vi "Convert API String Arguments to Data(variant).vi"(7 "Type":variant, 9 "error in (no error)":errorcluster, 11 "String":string) -> (1 "error":errorcluster, 3 "Data":variant)   [LabVIEW 2017, in "API String Arguments Support.lvlib"]
uses:
  API String Arguments Support.lvlib
  <vilib>/Utility/Data Type/Type Definitions/Data Type.ctl
  <userlib>/_NEVSTOP/Communicable State Machine(CSM)/AdvanceAPI/CSM - Keywords.vi
  <userlib>/_OpenG.lib/string/string.llb/Trim Whitespace (String Array)__ogtk.vi
  <vilib>/Utility/Data Type/NI_Data Type.lvlib
  <userlib>/_NEVSTOP/Communicable State Machine(CSM)/Communicable State Machine.lvlib
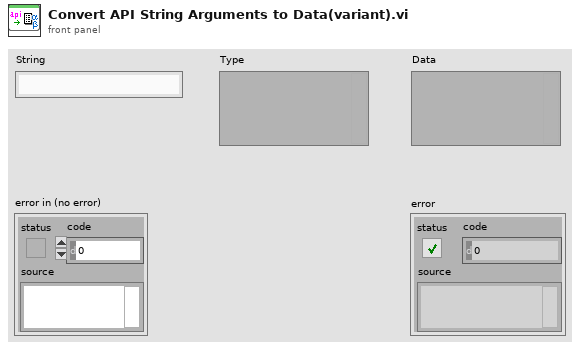
[diagram p1: front panel]
types:
  T1 = typedef "NI_Data Type.lvlib/Data Type.ctl" = enum8{"Invalid Type", "Void", "I8", "I16", "I32", "I64", "U8", "U16", "U32", "U64", "Single Float", "Double Float", "Extended Float", "Single Complex", "Double Complex", "Extended Complex", "Enum U8", "Enum U16", "Enum U32", "Enum U64", "Single Float With Unit", "Double Float With Unit", "Extended Float With Unit", "Single Complex with Unit", "Double Complex with Unit", "Extended Complex with Unit", "Boolean", "String", "Path", "Picture", "Tag", "Array", "Cluster", "Variant", "LV Variant", "Waveform", "Timestamp", "Digital Waveform", "Digital Data", "ExpressData", "Refnum", "External Data", "VI", "Poly VI", "LabVIEW Class Instance", "Fixed Point"}
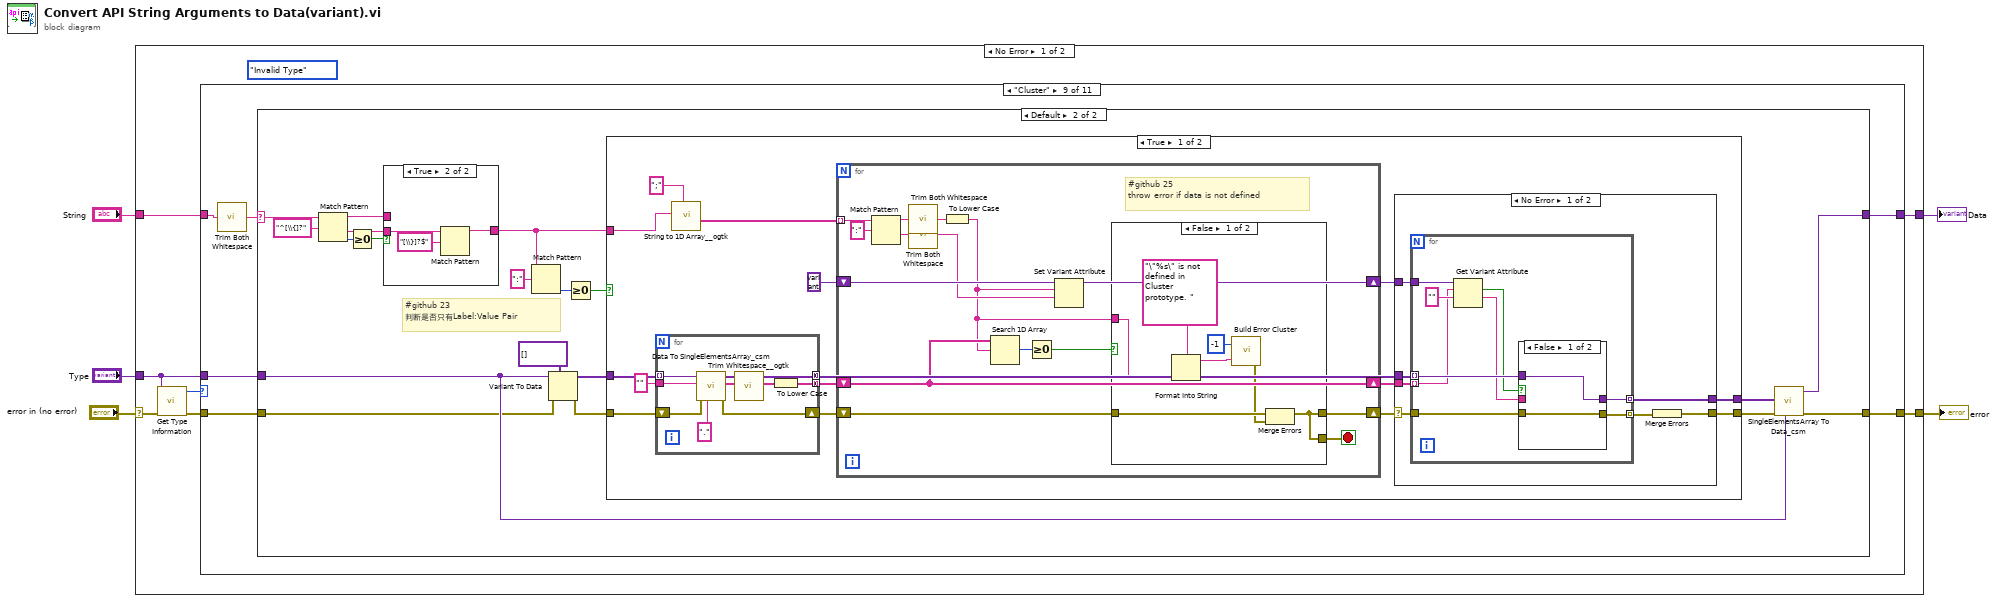
[diagram p0: block diagram]
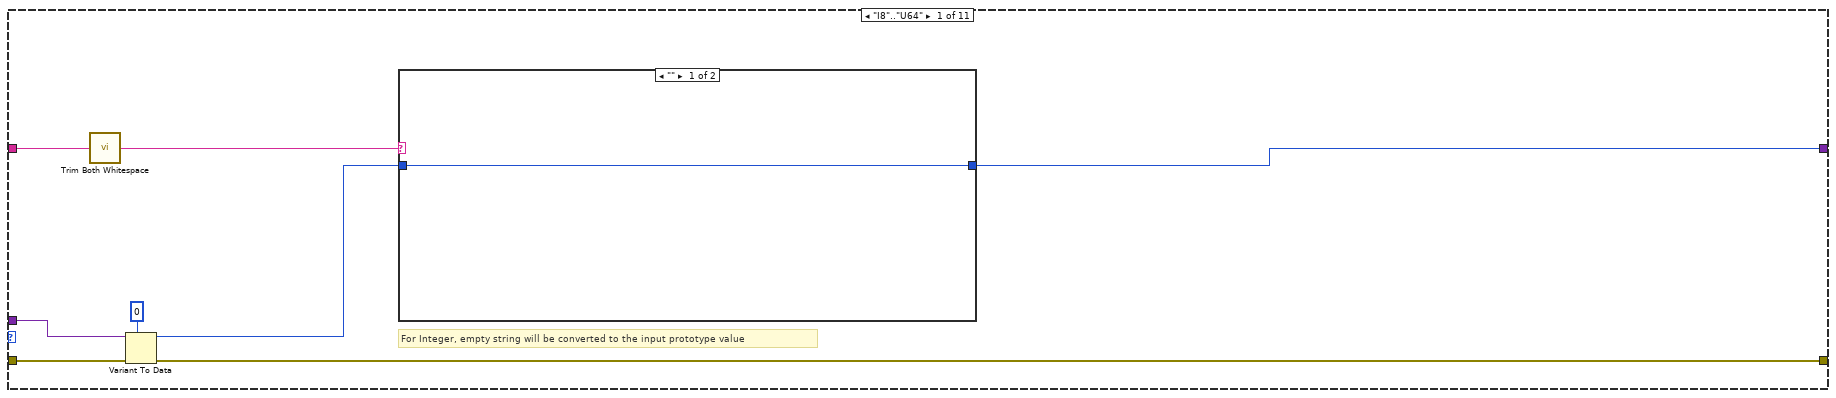
[diagram p2: hidden frame]
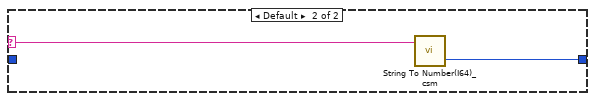
[diagram p3: hidden frame]
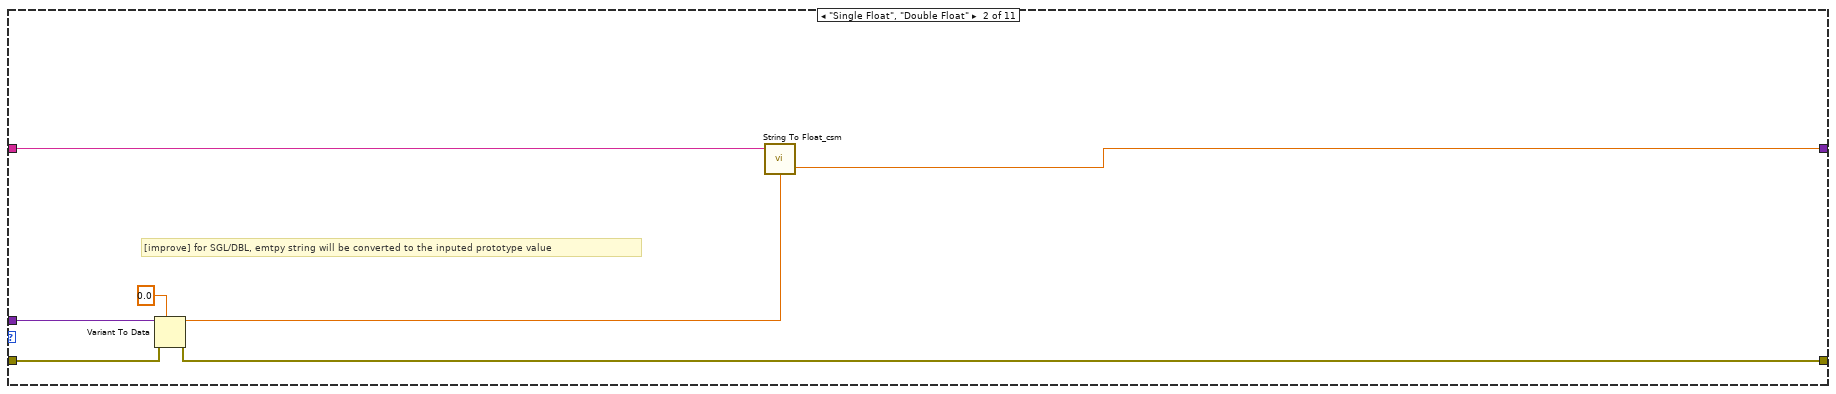
[diagram p4: hidden frame]
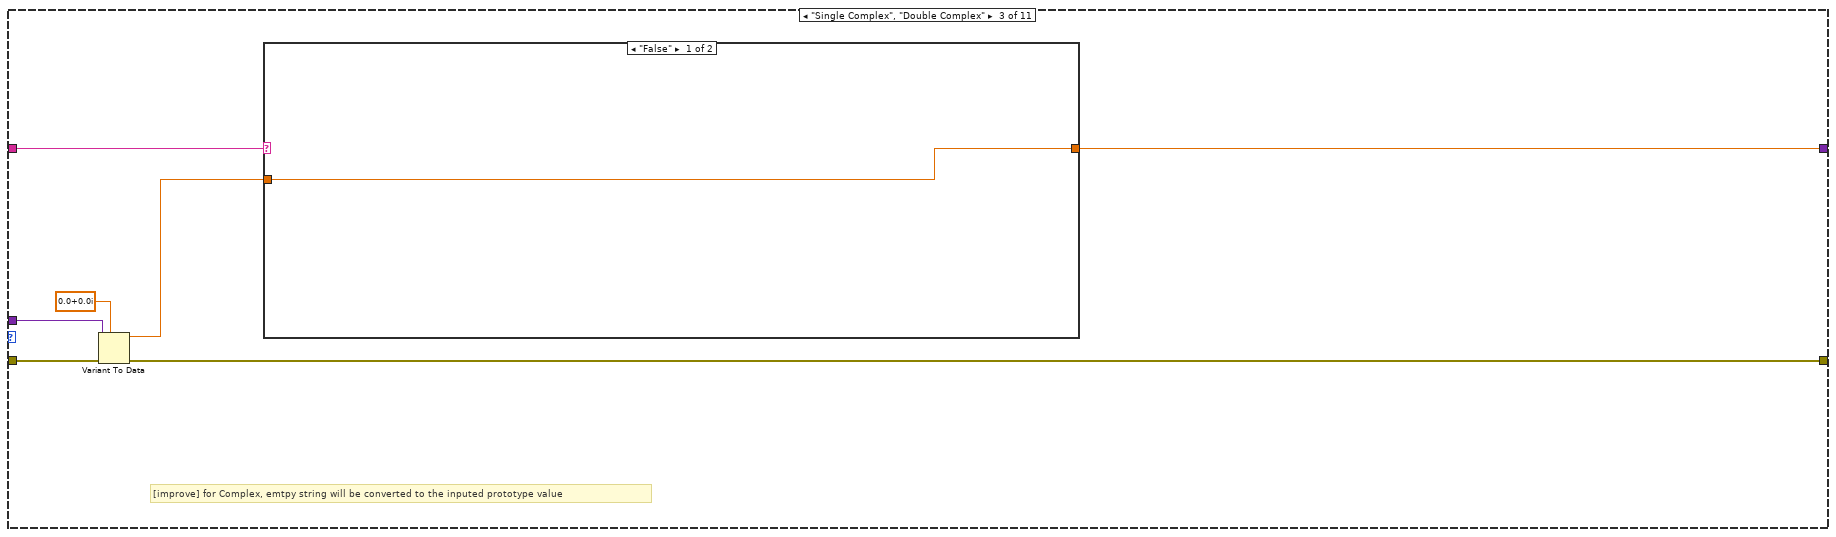
[diagram p5: hidden frame]
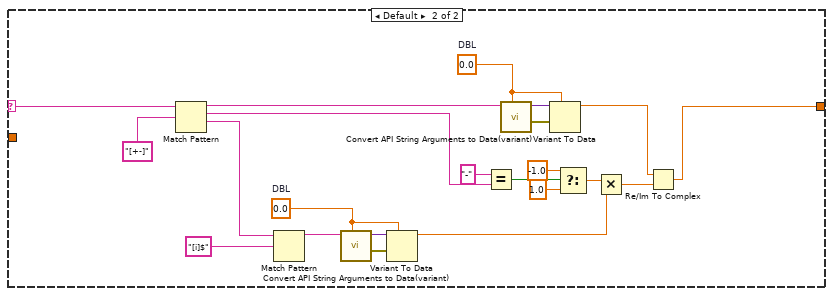
[diagram p6: hidden frame]
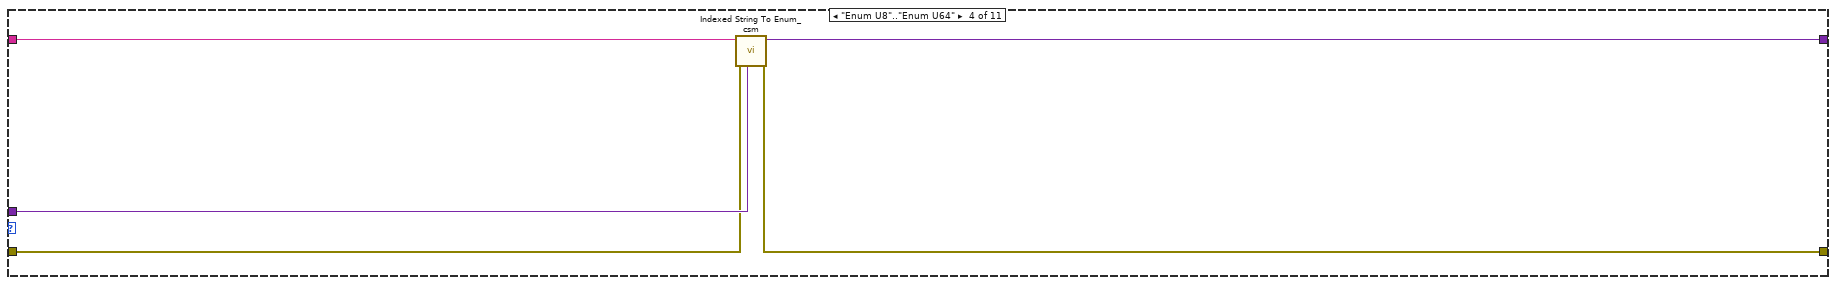
[diagram p7: hidden frame]
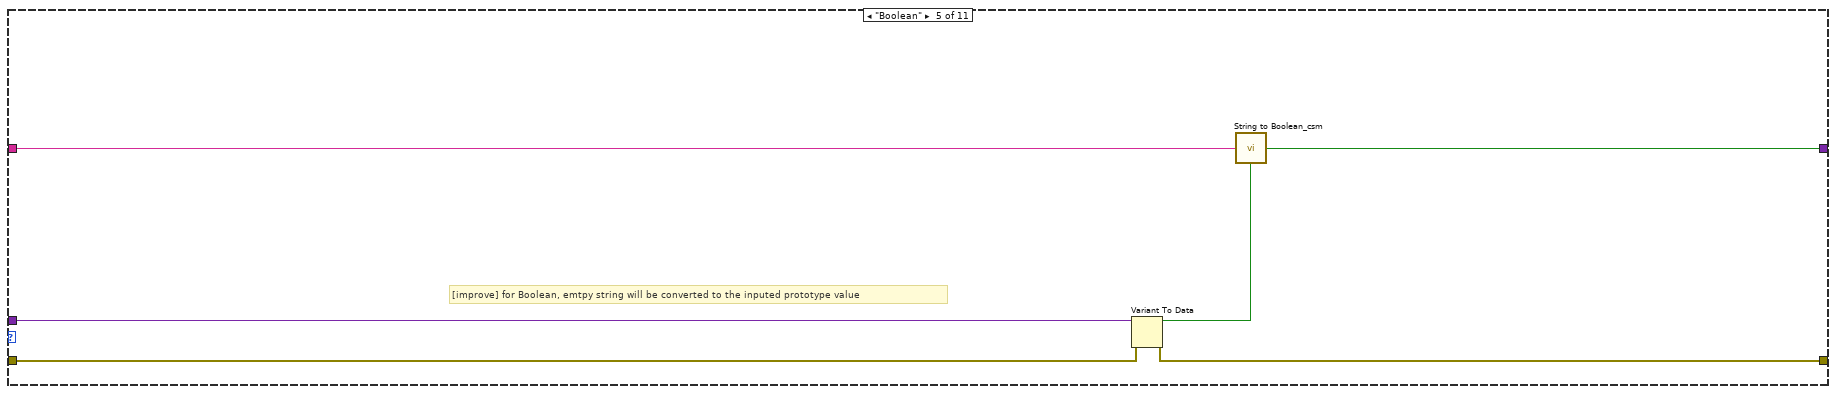
[diagram p8: hidden frame]
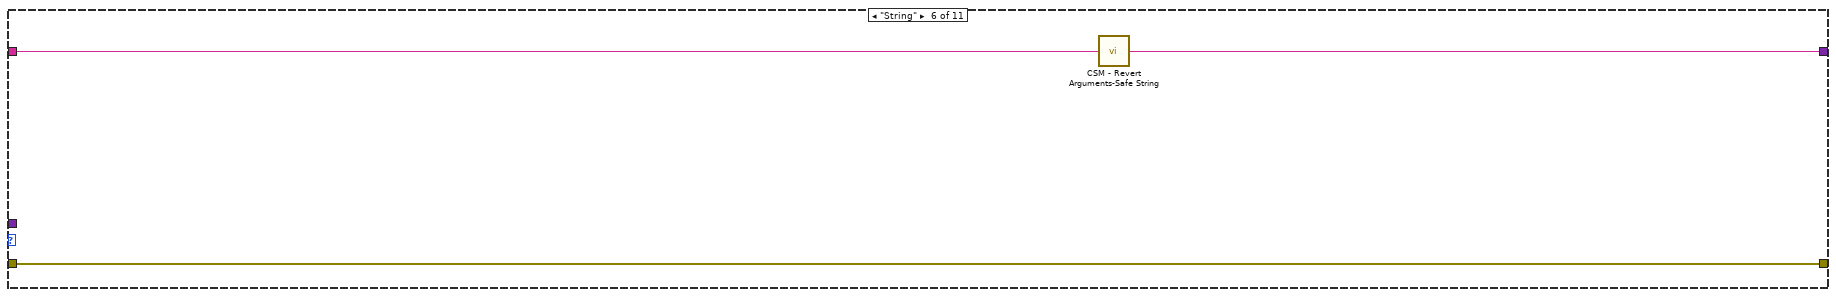
[diagram p9: hidden frame]
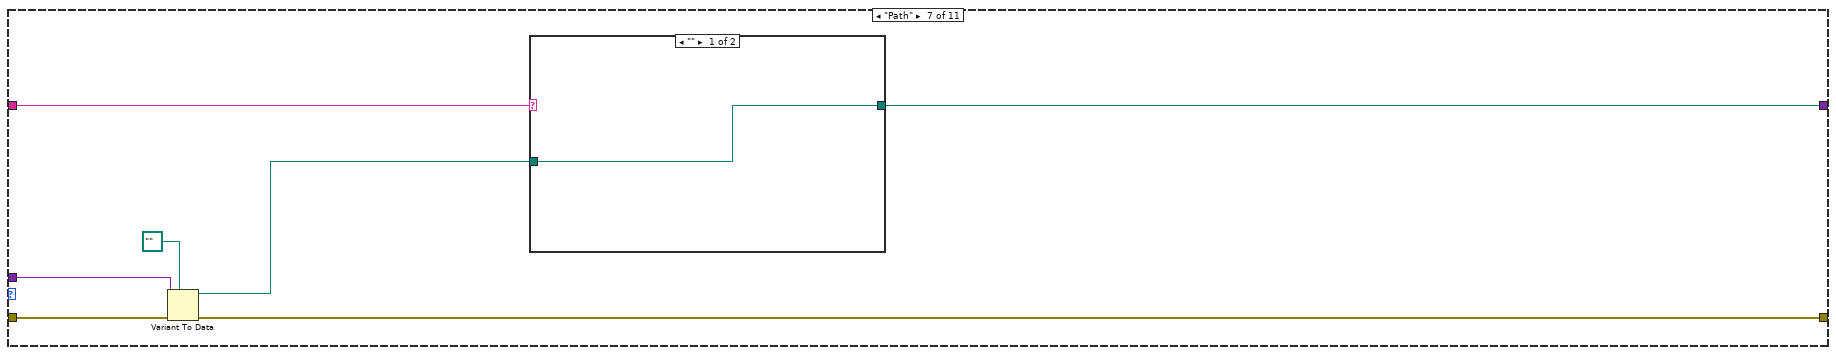
[diagram p10: hidden frame]
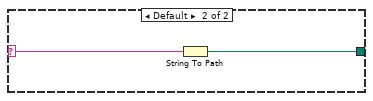
[diagram p11: hidden frame]
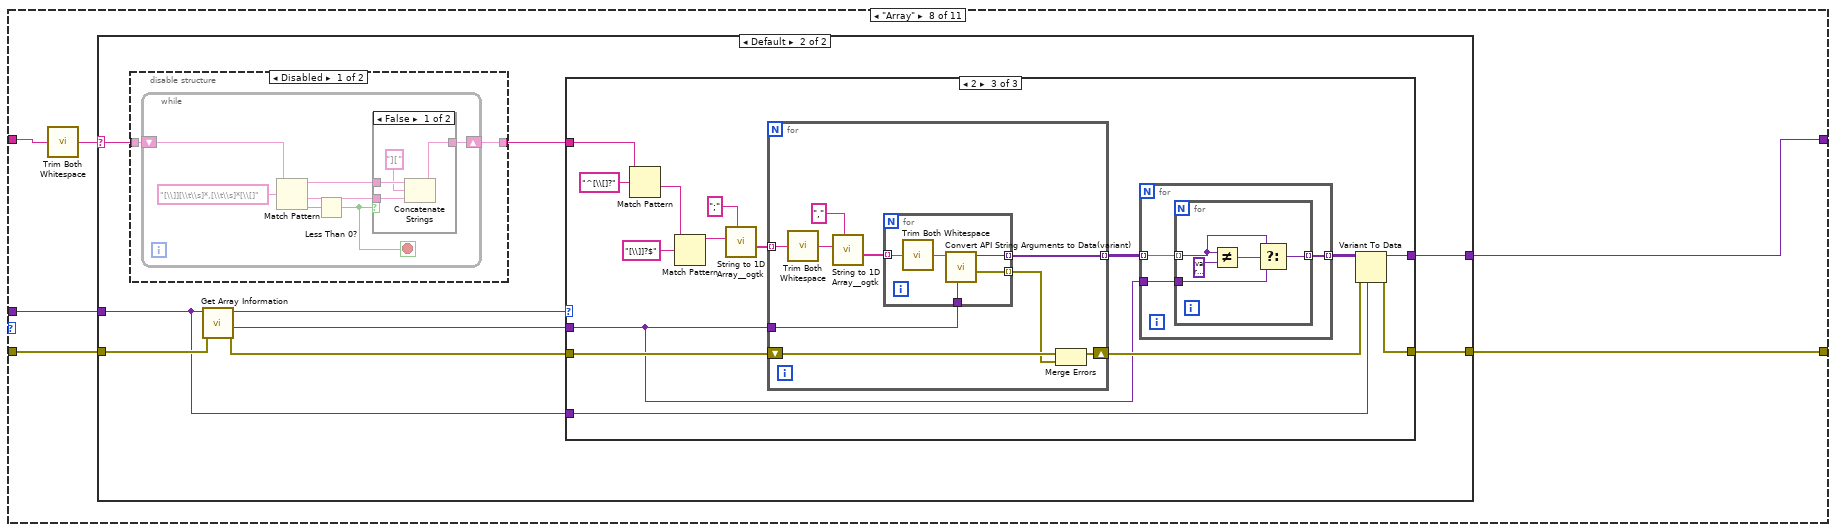
[diagram p12: hidden frame]
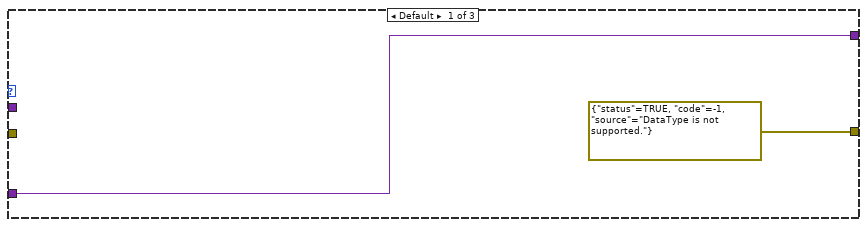
[diagram p16: hidden frame]
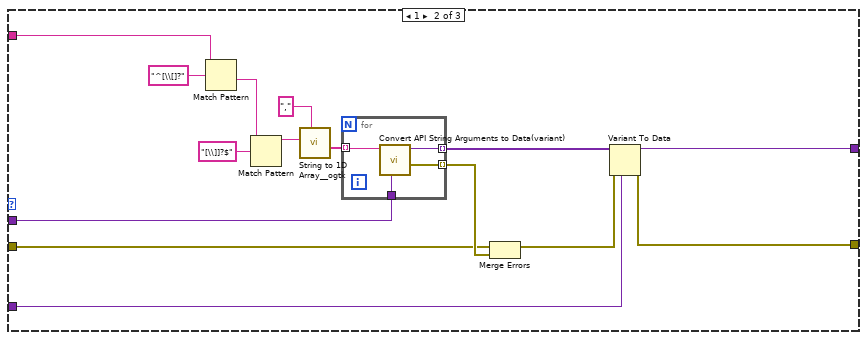
[diagram p17: hidden frame]
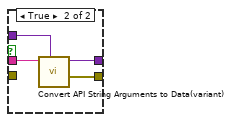
[diagram p19: hidden frame]
diagram:
  n1 = case shown="No Error" "error in (no error)" {
    selector: "error in (no error)" -> [w6 w340]
    tunnel: [w10 w340] -> w5
    tunnel: [w9 w339] -> w4
    tunnel: "Type" -> [w8 w339]
    tunnel: "String" -> [w7 _]
    frame No Error {
      (unwired) Data_Type."Invalid Type" ("type")
      n2 = call <vilib>:"Get Type Information.vi"("error in (no error)"=w6, "Variant"=w8) -> ("error out"=w11:errorcluster, "Type"=w12:T1)  [unwired: 5 in, 3 out]
      n3 = case shown="\"Cluster\"" w12 {
        tunnel: w11 -> [w18 w30 w37 w63 w67 w74 w81 w90 w176 w299 w304]
        tunnel: [w16 w27 w34 w62 w66 w74 w78 w88 w180 w296 w302] -> w10
        tunnel: [w19 w28 w35 w61 w70 w72 w79 w89 w179 w297 w303] -> w9
        tunnel: w8 -> [w14 w26 w33 w64 w69 _ w77 w87 w177 _ _]
        tunnel: w7 -> [w20 w29 w36 w65 w71 w73 w80 w86 w178 w298 w301]
        frame "I8".."U64" {
          # "For Integer, empty string will be converted to the input prototype value"
          n4 = call <userlib>:"Trim Both Whitespace.vi"("string"=w20) -> ("trimmed string"=w17:string)  [unwired: 1 in]
          n5 = Variant To Data(error in=w18, type=i64 0 ("64bit integer"), Variant=w14) -> (data=w13:i64, error out=w16:errorcluster)
          n6 = case shown="\"\"" w17 {
            selector: w17 -> [_ w22]
            tunnel: [w21 w23] -> w19
            tunnel: w13 -> [w21 _]
            frame "" {
            }
            frame Default {
              n7 = call "String To Number(I64)_csm.vi"("String"=w22) -> ("Numeric(I64)"=w23:i64)  [unwired: 4 in]
            }
          }
        }
        frame "Single Float", "Double Float" {
          # "[improve] for SGL/DBL, emtpy string will be converted to the inputed prototype value"
          n8 = Variant To Data(error in=w30, type=0.0 ("Default(0)"), Variant=w26) -> (data=w24:dbl, error out=w27:errorcluster)
          n9 = call "String To Float_csm.vi"("Default(0)"=w24, "String"=w29) -> ("Float"=w28:dbl)  [unwired: 3 in]
        }
        frame "Single Complex", "Double Complex" {
          # "[improve] for Complex, emtpy string will be converted to the inputed prototype value"
          n10 = Variant To Data(error in=w37, type=cdb 0.0+0.0i ("x + iy"), Variant=w33) -> (data=w31:cdb, error out=w34:errorcluster)
          n11 = case shown="\"False\"" w36 {
            selector: w36 -> [_ w59]
            tunnel: [w38 w39] -> w35
            tunnel: w31 -> [w38 _]
            frame "False" {
            }
            frame Default {
              w49 = 0.0  # DBL
              w52 = 0.0  # DBL
              n12 = Match Pattern(string=w59, regular expression="[+-]") -> (before substring=w56:string, match substring=w47:string, after substring=w58:string)  [unwired: 1 in, 1 out]
              n13 = Match Pattern(string=w58, regular expression="[i]$") -> (before substring=w55:string)  [unwired: 1 in, 3 out]
              n14 = call "Convert API String Arguments to Data(variant).vi"("Type"=w49, "String"=w55) -> ("error"=w51:errorcluster, "Data"=w50:variant)  [unwired: 8 in]
              n15 = Variant To Data(error in=w51, type=w49, Variant=w50) -> (data=w48:dbl)  [unwired: 1 out]
              n16 = Equal?(x="-", y=w47) -> (x = y?=w45:bool)
              n17 = call "Convert API String Arguments to Data(variant).vi"("Type"=w52, "String"=w56) -> ("error"=w54:errorcluster, "Data"=w53:variant)  [unwired: 8 in]
              n18 = Variant To Data(error in=w54, type=w52, Variant=w53) -> (data=w40:dbl)  [unwired: 1 out]
              n19 = Select(t=-1.0, s=w45, f=1.0 ("t")) -> (s? t:f=w44:dbl)
              n20 = Multiply(x=w44, y=w48) -> (x*y=w41:dbl)
              n21 = Re/Im To Complex(1:w41, 2:w40) -> (0:w39:cdb)
            }
          }
        }
        frame "Enum U8".."Enum U64" {
          n22 = call "Indexed String To Enum_csm.vi"("Variant"=w64, "error in (no error)"=w63, "String"=w65) -> ("error out"=w62:errorcluster, "Enum"=w61:variant)  [unwired: 7 in]
        }
        frame "Boolean" {
          # "[improve] for Boolean, emtpy string will be converted to the inputed prototype value"
          n23 = Variant To Data(error in=w67, Variant=w69) -> (data=w68:bool, error out=w66:errorcluster)  [unwired: 1 in]
          n24 = call "String to Boolean_csm.vi"("Default(F)"=w68, "String"=w71) -> ("Boolean"=w70:bool)  [unwired: 2 in]
        }
        frame "String" {
          n25 = call <userlib>:"CSM - Revert Arguments-Safe String.vi"("Safe Argurment String"=w73) -> ("Origin Argurment String"=w72:string)  [unwired: 8 in]
        }
        frame "Path" {
          n26 = Variant To Data(error in=w81, type=path "", Variant=w77) -> (data=w75:path, error out=w78:errorcluster)
          n27 = case shown="\"\"" w80 {
            selector: w80 -> [_ w84]
            tunnel: [w82 w83] -> w79
            tunnel: w75 -> [w82 _]
            frame "" {
            }
            frame Default {
              n28 = String To Path(string=w84) -> (path=w83:path)
            }
          }
        }
        frame "Array" {
          n29 = call <userlib>:"Trim Both Whitespace.vi"("string"=w86) -> ("trimmed string"=w85:string)  [unwired: 1 in]
          n30 = case shown="Default" w85 {
            selector: w85 -> [_ w93]
            tunnel: w90 -> [w92 w101]
            tunnel: [w91 w100] -> w89
            tunnel: [w92 w99] -> w88
            tunnel: w87 -> [w91 w95]
            frame "" {
            }
            frame Default {
              n31 = disable-structure shown="Disabled" {
                disable-tunnel: w93 -> [w103 w116]
                disable-tunnel: [w102 w116] -> w94
                frame Disabled {
                  n32 = while {
                    shift-right: [w106] -> w102
                    shift-left: w103 -> [w110]
                    stop <- w104 stop-if-true
                    n33 = Match Pattern(string=w110, regular expression="[\\]][\\t\\s]*,[\\t\\s]*[\\[]") -> (before substring=w108:string, after substring=w107:string, offset past match=w105:i32)  [unwired: 1 in, 1 out]
                    n34 = Less Than 0?(x=w105) -> (x < 0?=w104:bool)
                    n35 = case shown="False" w104 {
                      tunnel: w108 -> [w114 w115]
                      tunnel: w107 -> [w113 _]
                      tunnel: [w111 w115] -> w106
                      frame False {
                        n36 = Concatenate Strings(w114, "][" ("string"), w113) -> (w111:string)
                      }
                      frame True {
                      }
                    }
                  }
                }
                frame Enabled {
                }
              }
              n37 = call <vilib>:"Get Array Information.vi"("error in (no error)"=w101, "Variant"=w95) -> ("error out"=w98:errorcluster, "Array Element Data Type"=w97:variant, "Number of Dimensions"=w96:i32)  [unwired: 6 in, 1 out]
              n38 = case shown="2" w96 {
                tunnel: w94 -> [_ w133 w140]
                tunnel: [w118 w125 w152] -> w100
                tunnel: [errorcluster {"status"=TRUE, "code"=-1, "source"="DataType is not supported."} ("error out") w123 w150] -> w99
                tunnel: w98 -> [_ w122 w149]
                tunnel: w97 -> [_ w121 w144]
                tunnel: w95 -> [w118 w119 w147]
                frame Default {
                }
                frame 1 {
                  n39 = Match Pattern(string=w133, regular expression="^[\\[]?") -> (after substring=w130:string)  [unwired: 1 in, 3 out]
                  n40 = Match Pattern(string=w130, regular expression="[\\]]?$") -> (before substring=w129:string)  [unwired: 1 in, 3 out]
                  n41 = call <userlib>:"String to 1D Array__ogtk.vi"("delimiter (Tab)"=",", "string"=w129) -> ("Array of Strings"=w127:string[])  [unwired: 9 in]
                  n42 = for {
                    tunnel: w127 -> [w134] mode=indexing
                    tunnel: [w136] -> w126 mode=indexing
                    tunnel: [w135] -> w120 mode=indexing
                    tunnel: w121 -> [w137]
                    n43 = call "Convert API String Arguments to Data(variant).vi"("Type"=w137, "String"=w134) -> ("error"=w136:errorcluster, "Data"=w135:variant)  [unwired: 8 in]
                  }
                  n44 = Merge Errors(w122, w126) -> (w124:errorcluster)
                  n45 = Variant To Data(error in=w124, type=w119, Variant=w120) -> (data=w125:variant, error out=w123:errorcluster)
                }
                frame 2 {
                  n46 = Match Pattern(string=w140, regular expression="^[\\[]?") -> (after substring=w141:string)  [unwired: 1 in, 3 out]
                  n47 = Match Pattern(string=w141, regular expression="[\\]]?$") -> (before substring=w139:string)  [unwired: 1 in, 3 out]
                  n48 = call <userlib>:"String to 1D Array__ogtk.vi"("delimiter (Tab)"=";", "string"=w139) -> ("Array of Strings"=w138:string[])  [unwired: 9 in]
                  n49 = for {
                    tunnel: [w159] -> w146 mode=indexing
                    tunnel: w144 -> [w158]
                    shift-right: [w161] -> w151
                    shift-left: w149 -> [w160]
                    tunnel: w138 -> [w154] mode=indexing
                    n50 = call <userlib>:"Trim Both Whitespace.vi"("string"=w154) -> ("trimmed string"=w153:string)  [unwired: 1 in]
                    n51 = call <userlib>:"String to 1D Array__ogtk.vi"("delimiter (Tab)"=",", "string"=w153) -> ("Array of Strings"=w156:string[])  [unwired: 9 in]
                    n52 = for {
                      tunnel: w156 -> [w163] mode=indexing
                      tunnel: [w165] -> w155 mode=indexing
                      tunnel: [w164] -> w159 mode=indexing
                      tunnel: w158 -> [w166]
                      n53 = call <userlib>:"Trim Both Whitespace.vi"("string"=w163) -> ("trimmed string"=w162:string)  [unwired: 1 in]
                      n54 = call "Convert API String Arguments to Data(variant).vi"("Type"=w166, "String"=w162) -> ("error"=w165:errorcluster, "Data"=w164:variant)  [unwired: 8 in]
                    }
                    n55 = Merge Errors(w160, w155) -> (w161:errorcluster)
                  }
                  n56 = for {
                    tunnel: w146 -> [w169] mode=indexing
                    tunnel: [w168] -> w145 mode=indexing
                    tunnel: w144 -> [w167]
                    n57 = for {
                      tunnel: w169 -> [w171] mode=indexing
                      tunnel: [w170] -> w168 mode=indexing
                      tunnel: w167 -> [w172]
                      n58 = Not Equal?(x=w171, y=variant ("Data")) -> (x != y?=w173:bool)
                      n59 = Select(t=w171, s=w173, f=w172) -> (s? t:f=w170:variant)
                    }
                  }
                  n60 = Variant To Data(error in=w151, type=w147, Variant=w145) -> (data=w152:variant, error out=w150:errorcluster)
                }
              }
            }
          }
        }
        frame "Cluster" {
          n61 = call <userlib>:"Trim Both Whitespace.vi"("string"=w178) -> ("trimmed string"=w175:string)  [unwired: 1 in]
          n62 = case shown="Default" w175 {
            selector: w175 -> [_ w195]
            tunnel: [w181 w200] -> w180
            tunnel: [w182 w198] -> w179
            tunnel: w177 -> [w182 w190]
            tunnel: w176 -> [w181 w189]
            frame "" {
            }
            frame Default {
              # "#github 23\n判断是否只有Label:Value Pair"
              n63 = Match Pattern(string=w195, regular expression="^[\\{]?") -> (before substring=w192:string, after substring=w197:string, offset past match=w194:i32)  [unwired: 1 in, 1 out]
              n64 = Greater Or Equal To 0?(x=w194) -> (x >= 0?=w193:bool)
              n65 = case shown="True" w193 {
                tunnel: w197 -> [_ w294]
                tunnel: [w291 w292] -> w185
                tunnel: w192 -> [w291 _]
                frame False {
                }
                frame True {
                  n66 = Match Pattern(string=w294, regular expression="[\\}]?$") -> (before substring=w292:string)  [unwired: 1 in, 3 out]
                }
              }
              n67 = Match Pattern(string=w185, regular expression=":") -> (offset past match=w184:i32)  [unwired: 1 in, 3 out]
              n68 = Variant To Data(error in=w189, type=variant[] [] ("Array"), Variant=w190) -> (data=w188:variant[], error out=w187:errorcluster)
              n69 = Greater Or Equal To 0?(x=w184) -> (x >= 0?=w183:bool)
              n70 = case shown="True" w183 {
                tunnel: [w211 w273] -> w201
                tunnel: [w210 w274] -> w199
                tunnel: w188 -> [w208 w282]
                tunnel: w187 -> [w207 w281]
                tunnel: w185 -> [w206 w280]
                frame True {
                  n71 = for {
                    tunnel: [w247] -> w212 mode=concatenating
                    tunnel: [w241] -> w205 mode=concatenating
                    tunnel: "" ("parentUrl") -> [w244]
                    tunnel: w208 -> [w243] mode=indexing
                    shift-right: [w246] -> w203
                    shift-left: w207 -> [w249]
                    n72 = call "Data To SingleElementsArray_csm.vi"("Seperator(/)"=".", "error in (no error)"=w249, "parentUrl"=w244, "Cluster"=w243) -> ("error out"=w246:errorcluster, "Full NameList"=w245:string[], "DataElementArray"=w247:variant[])  [unwired: 5 in]
                    n73 = call-poly <userlib>:"Trim Whitespace__ogtk.vi"("String in"=w245) -> ("String out"=w242:string[])  [unwired: 6 in]
                    n74 = To Lower Case(string=w242) -> (all lower case string=w241:string[])
                  }
                  n75 = call <userlib>:"String to 1D Array__ogtk.vi"("delimiter (Tab)"=";", "string"=w206) -> ("Array of Strings"=w215:string[])  [unwired: 9 in]
                  n76 = for {
                    tunnel: w215 -> [w262] mode=indexing
                    shift-right: [w263] -> w213
                    shift-left: variant -> [w264]
                    shift-right: [w256] -> w204
                    shift-left: w205 -> [w256]
                    shift-right: [w253] -> w202
                    shift-left: w203 -> [w254]
                    stop <- w250 stop-if-true
                    # "#github 25\nthrow error if data is not defined"
                    n77 = Match Pattern(string=w262, regular expression=":") -> (before substring=w259:string, after substring=w260:string)  [unwired: 1 in, 2 out]
                    n78 = call <userlib>:"Trim Both Whitespace.vi"("string"=w259) -> ("trimmed string"=w257:string)  [unwired: 1 in]
                    n79 = call <userlib>:"Trim Both Whitespace.vi"("string"=w260) -> ("trimmed string"=w258:string)  [unwired: 1 in]
                    n80 = To Lower Case(string=w257) -> (all lower case string=w251:string)
                    n81 = Search 1D Array(1D array=w256, element=w251) -> (index of element=w255:i32)  [unwired: 1 in]
                    n82 = Greater Or Equal To 0?(x=w255) -> (x >= 0?=w252:bool)
                    n83 = Set Variant Attribute(Variant=w264, name=w251, value=w258) -> (Variant out=w263:variant)  [unwired: 1 in, 2 out]
                    n84 = case shown="False" w252 {
                      tunnel: w254 -> [w271 w272]
                      tunnel: [w265 w272] -> w253
                      tunnel: w251 -> [w266 _]
                      tunnel: [w265 _] -> w250
                      frame False {
                        n85 = Format Into String(format string="\"%s\" is not  defined in Cluster prototype. ", w266) -> (resulting string=w268:string)  [unwired: 2 in, 1 out]
                        n86 = call <userlib>:"Build Error Cluster.vi"("String to Prepend to source (\"\")"=w268, "code"=-1) -> ("error out"=w270:errorcluster)
                        n87 = Merge Errors(w271, w270) -> (w265:errorcluster)
                      }
                      frame True {
                      }
                    }
                  }
                  n88 = case shown="No Error" w202 {
                    selector: w202 -> [w217 w240]
                    tunnel: w213 -> [w223 _]
                    tunnel: w212 -> [w222 w239]
                    tunnel: [w220 w239] -> w211
                    tunnel: [w219 w240] -> w210
                    tunnel: w204 -> [w218 _]
                    frame No Error {
                      n89 = for {
                        tunnel: w223 -> [w232]
                        tunnel: w222 -> [w230] mode=indexing
                        tunnel: w217 -> [w225]
                        tunnel: w218 -> [w224] mode=indexing
                        tunnel: [w228] -> w220 mode=indexing
                        tunnel: [w227] -> w221 mode=indexing
                        n90 = Get Variant Attribute(Variant=w232, name=w224, default value (empty Variant)="" ("regular expression")) -> (found=w226:bool, value=w229:string)  [unwired: 1 in, 2 out]
                        n91 = case shown="False" w226 {
                          tunnel: w230 -> [w234 w238]
                          tunnel: w229 -> [_ w235]
                          tunnel: [w234 w237] -> w228
                          tunnel: [w233 w236] -> w227
                          tunnel: w225 -> [w233 _]
                          frame False {
                          }
                          frame True {
                            n92 = call "Convert API String Arguments to Data(variant).vi"("Type"=w238, "String"=w235) -> ("error"=w236:errorcluster, "Data"=w237:variant)  [unwired: 8 in]
                          }
                        }
                      }
                      n93 = Merge Errors(w221) -> (w219:errorcluster)
                    }
                    frame Error {
                    }
                  }
                }
                frame False {
                  w275 = 0 ("index")
                  # "#github 23\n如果没有发现Label:Value Pair\n将String转换为第一个基础类型"
                  n94 = for {
                    tunnel: [w288] -> w277 mode=concatenating
                    tunnel: [w286] -> _ mode=concatenating
                    tunnel: "" ("parentUrl") -> [w285]
                    tunnel: w282 -> [w284] mode=indexing
                    shift-right: [w287] -> w278
                    shift-left: w281 -> [w290]
                    n95 = call "Data To SingleElementsArray_csm.vi"("Seperator(/)"=".", "error in (no error)"=w290, "parentUrl"=w285, "Cluster"=w284) -> ("error out"=w287:errorcluster, "Full NameList"=w286:string[], "DataElementArray"=w288:variant[])  [unwired: 5 in]
                  }
                  n96 = Index Array(array=w277, index=w275) -> (element=w279:variant)
                  n97 = call "Convert API String Arguments to Data(variant).vi"("Type"=w279, "error in (no error)"=w278, "String"=w280) -> ("error"=w274:errorcluster, "Data"=w276:variant)  [unwired: 7 in]
                  n98 = Replace Array Subset(array=w277, new element=w276, index=w275) -> (w273:variant[])
                }
              }
              n99 = call "SingleElementsArray To Data_csm.vi"("Pototype"=w190, "error in (no error)"=w199, "DataElementArray"=w201) -> ("error out"=w200:errorcluster, "Cluster"=w198:variant)  [unwired: 7 in]
            }
          }
        }
        frame Default {
          n100 = call <userlib>:"CSM - Convert HexStr to Data.vi"("HEX String"=w298) -> ("Variant"=w297:variant, "error out"=w295:errorcluster)  [unwired: 7 in]
          n101 = Merge Errors(w299, w295) -> (w296:errorcluster)
        }
        frame "Timestamp" {
          n102 = call <userlib>:"Trim Both Whitespace.vi"("string"=w301) -> ("trimmed string"=w300:string)  [unwired: 1 in]
          n103 = case shown="Default" w300 {
            selector: w300 -> [_ w310]
            tunnel: w304 -> [w305 w313]
            tunnel: [w306 w312] -> w303
            tunnel: [w305 w311] -> w302
            frame "" {
              # "For Timestamp, empty string will be converted to current time."
              n104 = Get Date/Time In Seconds() -> (seconds since 1Jan1904=w306:timestamp)
            }
            frame Default {
              n105 = Match Pattern(string=w310, regular expression="^[0-9a-fA-F]$") -> (offset past match=w308:i32)  [unwired: 1 in, 3 out]
              n106 = Greater Or Equal To 0?(x=w308) -> (x >= 0?=w307:bool)
              n107 = case shown="False" w307 {
                tunnel: w313 -> [w319 w338]
                tunnel: [w320 w337] -> w312
                tunnel: [w318 w336] -> w311
                tunnel: w310 -> [w323 w334]
                frame False {
                  n108 = Match Pattern(string=w323, regular expression="(") -> (before substring=w317:string, after substring=w316:string)  [unwired: 1 in, 2 out]
                  n109 = Match Pattern(string=w316, regular expression=")") -> (before substring=w315:string)  [unwired: 1 in, 3 out]
                  n110 = call <userlib>:"Trim Both Whitespace.vi"("string"=w315) -> ("trimmed string"=w314:string)  [unwired: 1 in]
                  n111 = case shown="\"\", \"UTC\"" w314 {
                    tunnel: w317 -> [w329 w333]
                    tunnel: w315 -> [w330 _]
                    tunnel: [w326 w332] -> w320
                    tunnel: w319 -> [w325 w331]
                    tunnel: [w324 w331] -> w318
                    frame Default {
                      w327 = timestamp(0 s since 1904-01-01) ("Time Stamp")
                      n112 = Scan From String(format string=w330, input string=w329, error in=w325, default 1=w327) -> (error out=w324:errorcluster, output 1=w328:timestamp)  [unwired: 1 in, 2 out]
                      n113 = Select(t=w327, s=w324, f=w328) -> (s? t:f=w326:timestamp)
                    }
                    frame "", "UTC" {
                      n114 = call <vilib>:"ISO8601 DateString to Timestamp.vi"("ISO8601 Date String"=w333) -> ("Timestamp"=w332:timestamp)  [unwired: 8 in, 2 out]
                    }
                  }
                }
                frame True {
                  n115 = call <userlib>:"CSM - Convert HexStr to Data.vi"("HEX String"=w334) -> ("Variant"=w337:variant, "error out"=w335:errorcluster)  [unwired: 7 in]
                  n116 = Merge Errors(w338, w335) -> (w336:errorcluster)
                }
              }
            }
          }
        }
      }
    }
    frame Error {
    }
  }
  "Data" <- w4
  "error" <- w5
